vi "ConfigureTheDeviceForPointMeasurement.vi"(0 "heidenhain":bool, 1 "?":T2, 2 "CtiotfIn":bool, 3 "AndorIn":bool, 4 "KoherasIn":bool, 5 "ScannerIn":bool, 6 "AndorIn 2":bool, 7 "error in":errorcluster) -> (24 "result":bool, 27 "error out":errorcluster)   [LabVIEW 2011]
uses:
  Utilities/controls/ctlSeqFNs_Koheras.ctl
  Utilities/controls/ctlSeqFNs_CTIOTF.ctl
  Utilities/controls/ctlSeqFNs_Scanner.ctl
  Utilities/controls/ctlSeqFNs_Andor.ctl
  Utilities/controls/ctlSeqFNs_Heidenhain.ctl
  Utilities/controls/ctlSeqFNs_PCDeviceInit.ctl
  Utilities/controls/ctlSeqFNs_AVTGuppy.ctl
  <vilib>/userDefined/High Color/IMAQdx.ctl
  Utilities/controls/ctlSeqFNs_Main.ctl
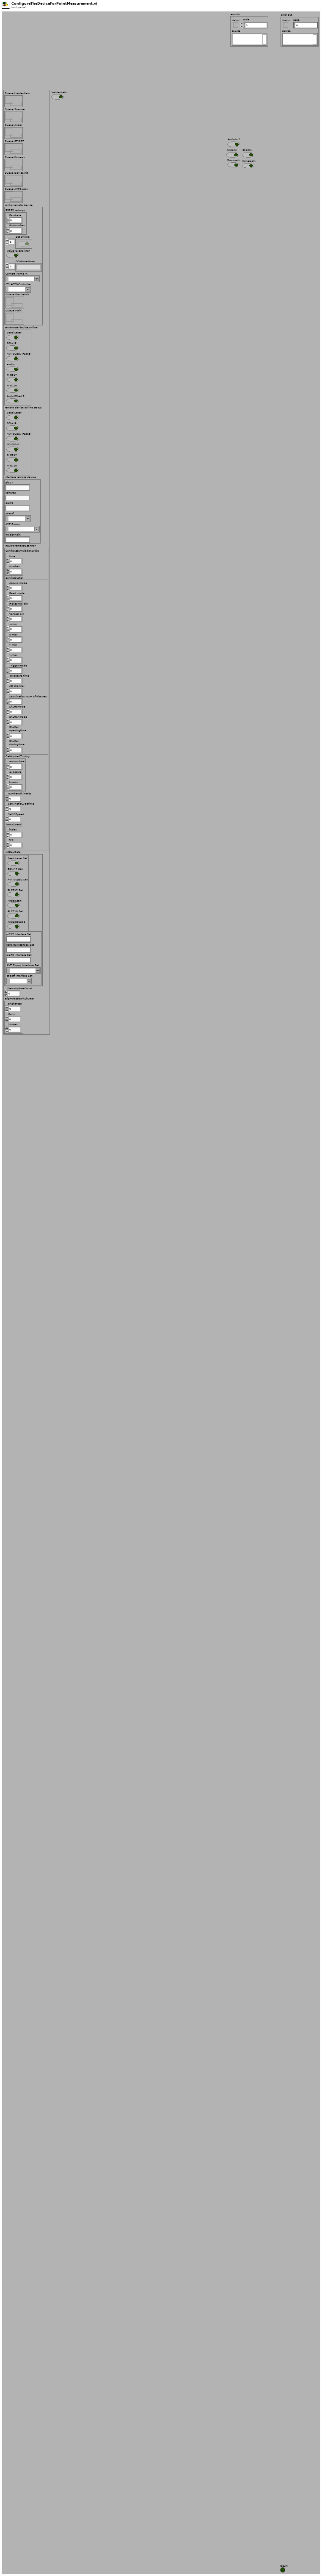
[diagram p1: front panel]
types:
  T1 = typedef "IMAQdx.ctl" = refnum<k21>
  T2 = cluster{"Queue Heidenhain":refnum<queue>, "Queue Scanner":refnum<queue>, "Queue Andor":refnum<queue>, "Queue CTIOTF":refnum<queue>, "Queue Koheras":refnum<queue>, "Queue DeviceInit":refnum<queue>, "Queue AVTGuppy":refnum<queue>, "config remote device":cluster{"RS232 settings":cluster{"Baudrate":u16, "Portnumber":i32}, "Set Online":bool[], "Value (Signaling)":bool, "COM-Interfaces":string[], "Camera Name In":T1, "CTI AOTF-Controller":refnum<visa-resource-name>, "Queue DeviceInit":refnum<queue>, "Queue Main":refnum<queue>}, "set remote device online":cluster{"Seed Laser":bool, "8Ch-HP":bool, "AVT Guppy F036B":bool, "andor":bool, "PI E517":bool, "PI E710":bool, "Andor2Start 2":bool}, "remote device online status":cluster{"Seed Laser":bool, "8Ch-HP":bool, "AVT Guppy F036B":bool, "ND-281-D":bool, "PI E517":bool, "PI E710":bool}, "interface remote device":cluster{"pi517":string, "koheras":string, "pie70":string, "ctiaotf":refnum<visa-resource-name>, "AVT Guppy":T1, "heidenhain":string}, "InputParameterScanner":cluster{"ConfigAccumulationCycle":cluster{"time":sgl, "number":i32}, "ConfigCluster":cluster{"Acquis. mode":u16, "Read mode":u16, "Horizontal bin":i32, "Vertical bin":i32, "x-min":i32, "x-max":i32, "y-min":i32, "y-max":i32, "Trigger mode":u16, " Exposure time":sgl, "AD channel":i32, "Set Kinetics, Num of Pictures":i32, "Shutter type":u16, "Shutter mode":u16, "Shutter\nopeningtime":i32, "Shutter\nclosingtime":i32}, "GetAquiredTiming":cluster{"accumulate":sgl, "exposure":sgl, "kinetic":sgl}, "NumberOfKinetics":i32, "SetKineticCycletime":sgl, "SetVSSpeed":i32, "SetHsSpeed":cluster{"index":i32, "typ":i32}}, "initDevData":cluster{cluster{"Seed Laser Set":bool, "8Ch-HP Set":bool, "AVT Guppy Set":bool, "PI E517 Set":bool, "AndorStart":bool, "PI E710 Set":bool, "Andor2Start 2":bool}, cluster{"pi517 Interface Set":string, "koheras Interface Set":string, "pie70 interface Set":string, "AVT Guppy Interface Set":T1, "ctiaotf interface Set":refnum<visa-resource-name>}}, "StatusUpdateCount":dbl, "BrightnessGainShutter":cluster{"Brightness":i32, "Gaiin":i32, "Shutter":i32}}
  T3 = typedef "ctlSeqFNs_Koheras.ctl" = enum16{"ERROR", "INIT", "Initialization", "Configuration", "Measurement", "Shutdown", "IDLE", "EXIT"}
  T4 = typedef "ctlSeqFNs_Heidenhain.ctl" = enum16{"ERROR", "INIT", "Initialization", "Configuration", "Measurement", "Shutdown", "IDLE", "EXIT"}
  T5 = typedef "ctlSeqFNs_CTIOTF.ctl" = enum16{"ERROR", "INIT", "Initialization", "Configuration", "Measurement", "Shutdown", "IDLE", "EXIT"}
  T6 = typedef "ctlSeqFNs_Scanner.ctl" = enum16{"ERROR", "INIT", "Initialization", "Configuration", "Measurement", "Shutdown", "IDLE", "EXIT"}
  T7 = typedef "ctlSeqFNs_Andor.ctl" = enum16{"ERROR", "INIT", "Initialization", "Configuration", "Measurement", "Shutdown", "IDLE", "EXIT"}
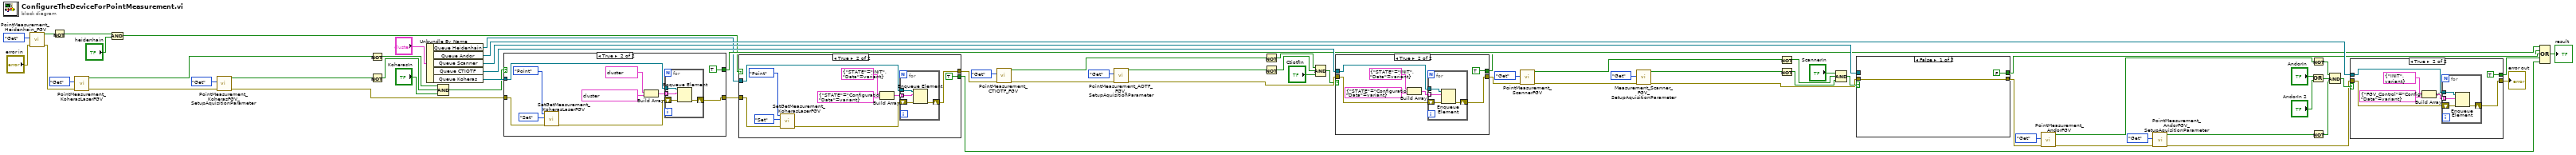
[diagram p0: block diagram]
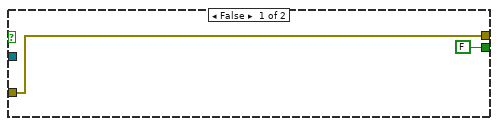
[diagram p2: hidden frame]
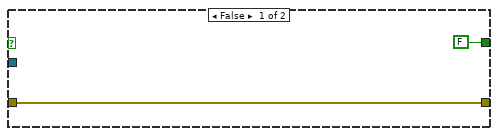
[diagram p3: hidden frame]
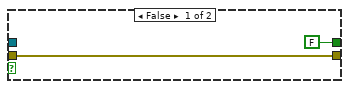
[diagram p4: hidden frame]
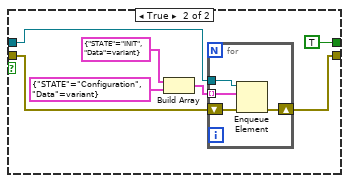
[diagram p5: hidden frame]
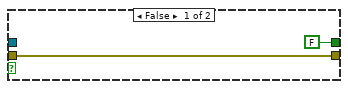
[diagram p6: hidden frame]
diagram:
  n1 = call "PointMeasurement_Heidenhain_FGV.vi"("error in"="error in", "Set_Get"=enum16{"Set", "Get"}."Get") -> ("error out"=w6:errorcluster, "Get"=w4:bool)  [unwired: 8 in]
  n2 = Not(x=w4) -> (.not. x?=w3:bool)
  n3 = call "PointMeasurement_KoherasLaserFGV.vi"("error in"=w6, "Set_Get"=enum16{"Set", "Get"}."Get") -> ("error out"=w54:errorcluster, "Get"=w52:bool)  [unwired: 8 in]
  n4 = Compound Arithmetic op=AND(w3, "heidenhain") -> (w1:bool)
  n5 = call "PointMeasurement_KoherasFGV_SetupAquisitionParameter.vi"("error in"=w54, "FGV_Control"=enum16{"Set", "Get"}."Get") -> ("error out"=w47:errorcluster, "Get"=w43:bool)  [unwired: 8 in]
  n6 = Not(x=w52) -> (.not. x?=w41:bool)
  n7 = Not(x=w43) -> (.not. x?=w40:bool)
  n8 = Unbundle By Name("?") -> ("Queue Heidenhain"=w11:refnum<queue>, "Queue Andor"=w62:refnum<queue>, "Queue Scanner"=w66:refnum<queue>, "Queue CTIOTF"=w65:refnum<queue>, "Queue Koheras"=w64:refnum<queue>)
  n9 = Compound Arithmetic op=AND(w41, w40, "KoherasIn") -> (w38:bool)
  n10 = case shown="True" w38 {
    tunnel: [w68 w78] -> w10
    tunnel: w64 -> [_ w77]
    tunnel: w47 -> [w68 w72]
    tunnel: [FALSE TRUE] -> w28
    frame False {
    }
    frame True {
      n11 = call "SetGetMeasurement_KoherasLaserFGV.vi"("error in"=w72, "FGV_Control"=enum16{"Set", "Get"}."Set", "MeasurementTypeIn"=enum16{"Point", "Linie"}."Point") -> ("error out"=w75:errorcluster)  [unwired: 7 in, 1 out]
      n12 = Build Array(cluster{"Data":variant, "FGV_Control":T3} {"Data"=variant, "FGV_Control"=enum."INIT"} ("element"), cluster{"Data":variant, "FGV_Control":T3} {"Data"=variant, "FGV_Control"=enum."Configuration"} ("element")) -> (w76:cluster{"Data":variant, "FGV_Control":T3}[])
      n13 = for {
        tunnel: w77 -> [w82]
        tunnel: w76 -> [w79] mode=indexing
        shift-right: [w81] -> w78
        shift-left: w75 -> [w80]
        n14 = Enqueue Element(queue=w82, element=w79, error in (no error)=w80) -> (error out=w81:errorcluster)  [unwired: 1 in, 2 out]
      }
    }
  }
  n15 = case shown="True" w1 {
    tunnel: [w84 w94] -> w9
    tunnel: w11 -> [_ w93]
    tunnel: w10 -> [w84 w88]
    tunnel: [FALSE TRUE] -> w8
    frame False {
    }
    frame True {
      n16 = call "SetGetMeasurement_KoherasLaserFGV.vi"("error in"=w88, "FGV_Control"=enum16{"Set", "Get"}."Set", "MeasurementTypeIn"=enum16{"Point", "Linie"}."Point") -> ("error out"=w91:errorcluster)  [unwired: 7 in, 1 out]
      n17 = Build Array(cluster{"STATE":T4, "Data":variant} {"STATE"=enum."INIT", "Data"=variant} ("element"), cluster{"STATE":T4, "Data":variant} {"STATE"=enum."Configuration", "Data"=variant} ("element")) -> (w92:cluster{"STATE":T4, "Data":variant}[])
      n18 = for {
        tunnel: w93 -> [w98]
        tunnel: w92 -> [w95] mode=indexing
        shift-right: [w97] -> w94
        shift-left: w91 -> [w96]
        n19 = Enqueue Element(queue=w98, element=w95, error in (no error)=w96) -> (error out=w97:errorcluster)  [unwired: 1 in, 2 out]
      }
    }
  }
  n20 = call "PointMeasurement_CTIOTF_FGV.vi"("error in"=w9, "Set_Get"=enum16{"Set", "Get"}."Get") -> ("error out"=w50:errorcluster, "Get"=w48:bool)  [unwired: 8 in]
  n21 = call "PointMeasurement_AOTF_FGV_SetupAquisitionParameter.vi"("error in"=w50, "FGV_Control"=enum16{"Set", "Get"}."Get") -> ("error out"=w51:errorcluster, "Get"=w42:bool)  [unwired: 8 in]
  n22 = Not(x=w48) -> (.not. x?=w37:bool)
  n23 = Not(x=w42) -> (.not. x?=w36:bool)
  n24 = Compound Arithmetic op=AND(w37, w36, "CtiotfIn") -> (w34:bool)
  n25 = case shown="True" w34 {
    tunnel: [w100 w107] -> w56
    tunnel: w51 -> [w100 w102]
    tunnel: w65 -> [_ w106]
    tunnel: [FALSE TRUE] -> w27
    frame False {
    }
    frame True {
      n26 = Build Array(cluster{"STATE":T5, "Data":variant} {"STATE"=enum."INIT", "Data"=variant} ("element"), cluster{"STATE":T5, "Data":variant} {"STATE"=enum."Configuration", "Data"=variant} ("element")) -> (w104:cluster{"STATE":T5, "Data":variant}[])
      n27 = for {
        tunnel: w106 -> [w111]
        tunnel: w104 -> [w108] mode=indexing
        shift-right: [w110] -> w107
        shift-left: w102 -> [w109]
        n28 = Enqueue Element(queue=w111, element=w108, error in (no error)=w109) -> (error out=w110:errorcluster)  [unwired: 1 in, 2 out]
      }
    }
  }
  n29 = call "PointMeasurement_ScannerFGV.vi"("error in"=w56, "Set_Get"=enum16{"Set", "Get"}."Get") -> ("error out"=w17:errorcluster, "Get"=w57:bool)  [unwired: 8 in]
  n30 = call "Measurement_Scanner_FGV_SetupAquisitionParameter.vi"("error in"=w17, "FGV_Control"=enum16{"Set", "Get"}."Get") -> ("error out"=w15:errorcluster, "Get"=w14:bool)  [unwired: 8 in]
  n31 = Not(x=w57) -> (.not. x?=w19:bool)
  n32 = Not(x=w14) -> (.not. x?=w13:bool)
  n33 = Compound Arithmetic op=AND("ScannerIn", w19, w13) -> (w18:bool)
  n34 = case shown="False" w18 {
    tunnel: w15 -> [w113 w120]
    tunnel: w66 -> [_ w119]
    tunnel: [w113 w118] -> w55
    tunnel: [FALSE TRUE] -> w26
    frame False {
    }
    frame True {
      n35 = Build Array(cluster{"STATE":T6, "Data":variant} {"STATE"=enum."INIT", "Data"=variant} ("element"), cluster{"STATE":T6, "Data":variant} {"STATE"=enum."Configuration", "Data"=variant} ("element")) -> (w116:cluster{"STATE":T6, "Data":variant}[])
      n36 = for {
        tunnel: w119 -> [w124]
        tunnel: w116 -> [w122] mode=indexing
        shift-right: [w123] -> w118
        shift-left: w120 -> [w121]
        n37 = Enqueue Element(queue=w124, element=w122, error in (no error)=w121) -> (error out=w123:errorcluster)  [unwired: 1 in, 2 out]
      }
    }
  }
  n38 = call "PointMeasurement_AndorFGV.vi"("error in"=w55, "Set_Get"=enum16{"Set", "Get"}."Get") -> ("error out"=w44:errorcluster, "Get"=w45:bool)  [unwired: 8 in]
  n39 = call "PointMeasurement_AndorFGV_SetupAquisitionParameter.vi"("error in"=w44, "FGV_Control"=enum16{"Set", "Get"}."Get") -> ("error out"=w29:errorcluster, "Get"=w32:bool)  [unwired: 8 in]
  n40 = Not(x=w45) -> (.not. x?=w31:bool)
  n41 = Or(x="AndorIn", y="AndorIn 2") -> (x .or. y?=w22:bool)
  n42 = Not(x=w32) -> (.not. x?=w30:bool)
  n43 = Compound Arithmetic op=AND(w31, w22, w30) -> (w33:bool)
  n44 = case shown="True" w33 {
    tunnel: w29 -> [w126 w127]
    tunnel: [w126 w133] -> w63
    tunnel: w62 -> [_ w132]
    tunnel: [FALSE TRUE] -> w25
    frame False {
    }
    frame True {
      n45 = Build Array(cluster{"FGV_Control":T7, "Data":variant} {"FGV_Control"=enum."INIT", "Data"=variant} ("element"), cluster{"FGV_Control":T7, "Data":variant} {"FGV_Control"=enum."Configuration", "Data"=variant} ("element")) -> (w130:cluster{"FGV_Control":T7, "Data":variant}[])
      n46 = for {
        tunnel: w132 -> [w137]
        tunnel: w130 -> [w135] mode=indexing
        shift-right: [w136] -> w133
        shift-left: w127 -> [w134]
        n47 = Enqueue Element(queue=w137, element=w135, error in (no error)=w134) -> (error out=w136:errorcluster)  [unwired: 1 in, 2 out]
      }
    }
  }
  "error out" <- w63
  n48 = Compound Arithmetic op=OR(w28, w27, w26, w25, w8) -> (→"result":bool)
